vi "校准专用.vi"() -> ()   [LabVIEW 2021]
uses:
  <vilib>/Utility/file.llb/Write Delimited Spreadsheet (DBL).vi
  <vilib>/addons/_NISVFA/_Generation/SoundVib_Generation.lvlib
panel:
  in  "功能选定":u16(ring)=3 items=["保存 10K校准文件", "保存 20K校准文件", "保存 20K无样品文件", "不保存任何文件"]
  out "Time waveform 3":waveform(dbl)(graph)
  out "Time waveform 1":waveform(dbl)(graph)
  out "Time waveform 2":waveform(dbl)(graph)
  out "Time waveform 4":waveform(dbl)(graph)
  in  "开始测量":bool
  in  "停止频率（Hz）":dbl=20000.0 format="%#.2f"
  in  "幅值（V）":dbl=0.1 format="%.3f"
  in  "开始频率（Hz）":dbl=10.0 format="%#.2f"
  # "数据格式：9位小数精度"
  # "注意：\n请确认功能选择正确！\n请把原有文件做好备份再开始测量！新文件会覆盖原有文件。"
  # "扫频激励参数"
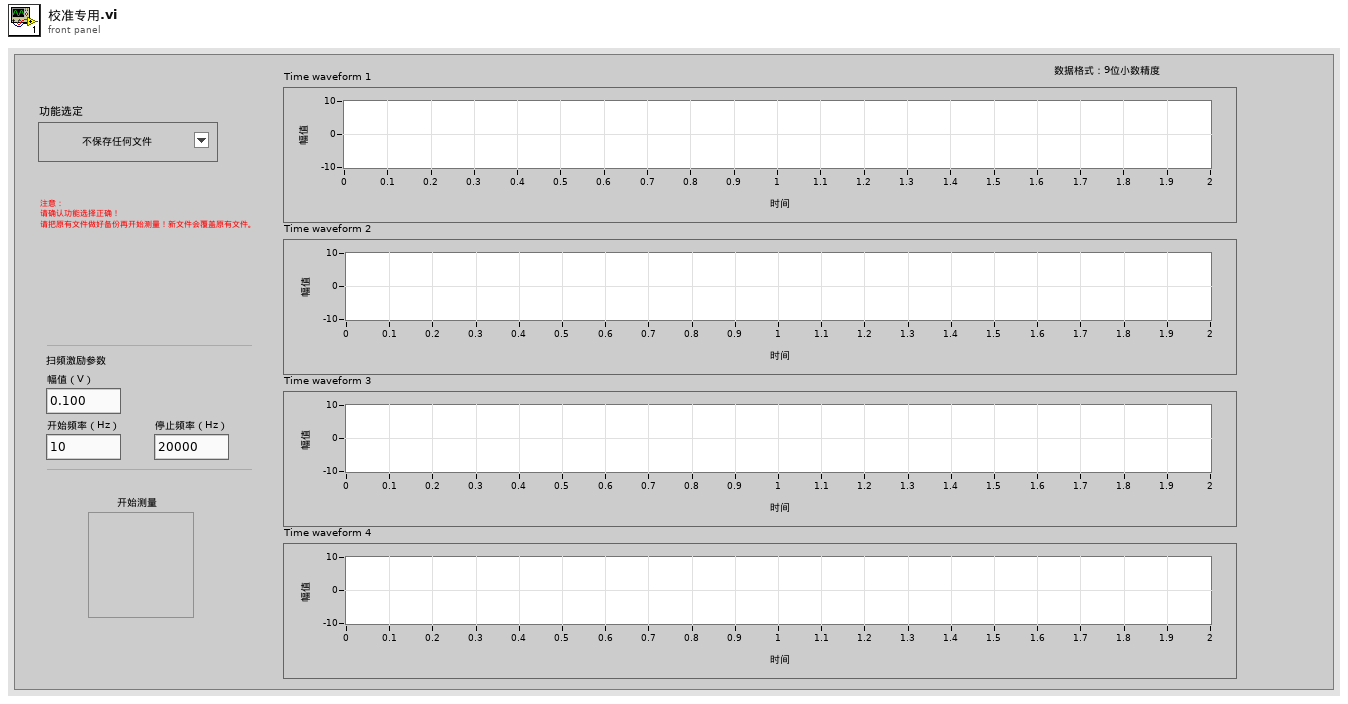
[diagram p1: front panel]
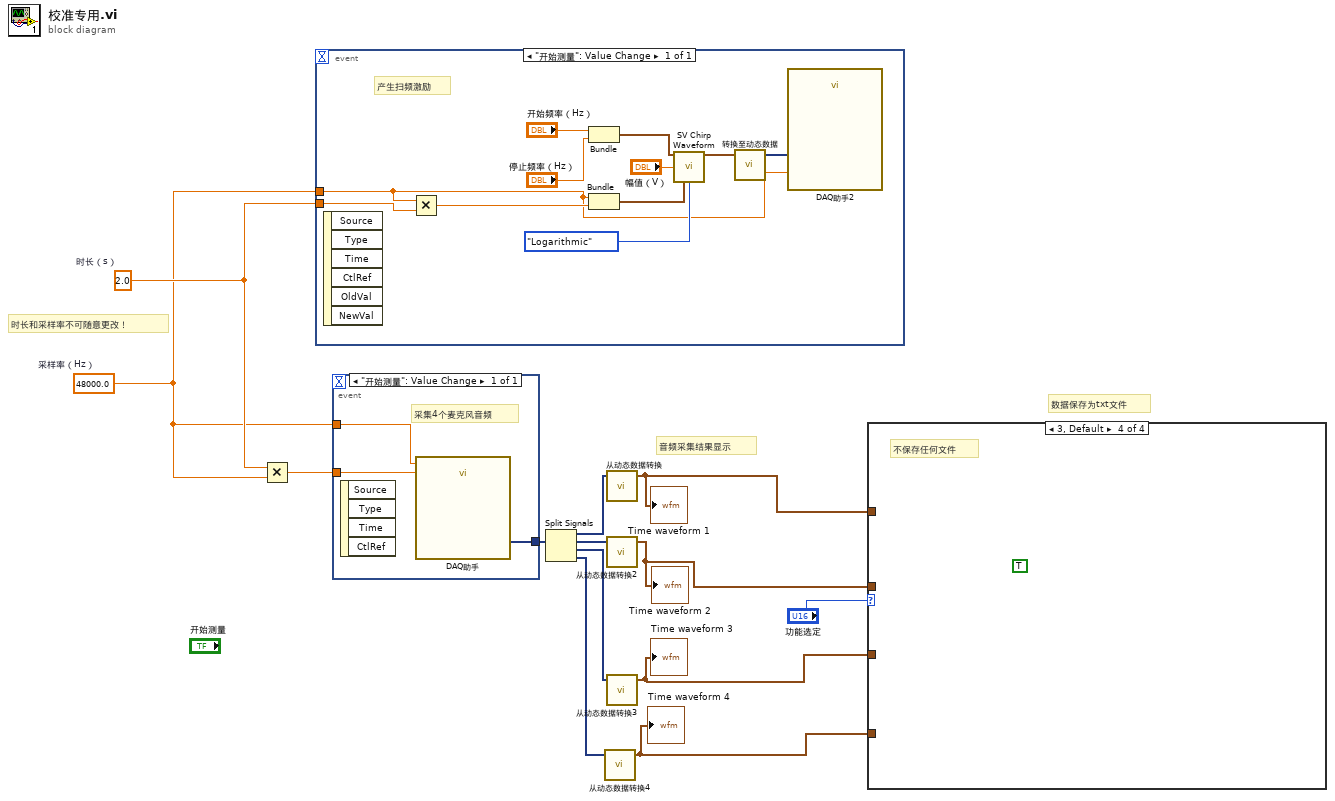
[diagram p0: block diagram]
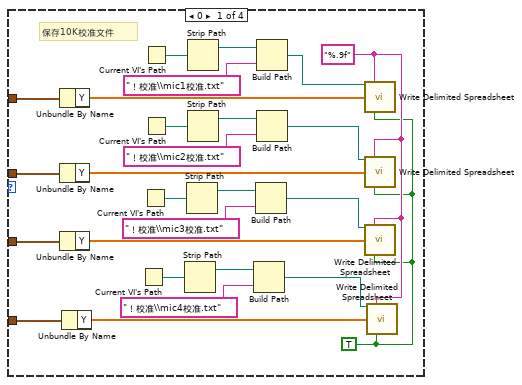
[diagram p2: hidden frame]
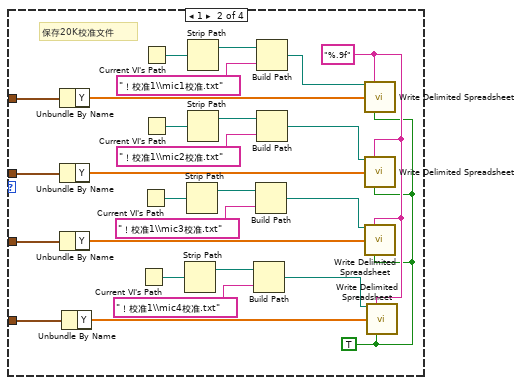
[diagram p3: hidden frame]
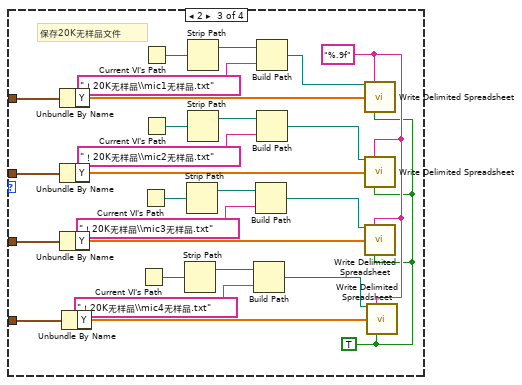
[diagram p4: hidden frame]
diagram:
  w7 = 48000.0  # 采样率（Hz）
  w12 = 2.0  # 时长（s）
  # "数据保存为txt文件"
  # "时长和采样率不可随意更改！"
  # "音频采集结果显示"
  n1 = Multiply(x=w12, y=w7) -> (x*y=w13:dbl)
  n2 = event shown="[0] \"开始测量\": Value Change" {
    selector: _ -> [_]
    dyn-events: _ -> [_]
    timeout: _ -> [_]
    tunnel: w12 -> [w24]
    tunnel: w7 -> [w14]
    event "开始测量": Value Change {
      # "产生扫频激励"
      n3 = event-data() -> ()  [unwired: 1 in, 6 out]
      n4 = Multiply(x=w14, y=w24) -> (x*y=w23:dbl)
      n5 = Bundle("开始频率（Hz）"="开始频率（Hz）", "停止频率（Hz）"="停止频率（Hz）") -> (w16:cluster{"开始频率（Hz）":dbl, "停止频率（Hz）":dbl})  [unwired: 1 in]
      n6 = Bundle("采样率（Hz）"=w14, w23) -> (w21:cluster{"采样率（Hz）":dbl, dbl})  [unwired: 1 in]
      n7 = call <vilib>:"SV Chirp Waveform.vi"("frequency range"=w16, "amplitude"="幅值（V）", "sampling info"=w21, "frequency spacing"=enum16{"Linear", "Logarithmic"}."Logarithmic") -> ("chirp signal"=w22:waveform(dbl))  [unwired: 9 in, 2 out]
      n8 = call "转换至动态数据"("Waveform"=w22) -> ("Dynamic Data Type"=w15:dynamicdata)  [unwired: 3 in]
      n9 = call "DAQ助手2"("data"=w15, "速率"=w14) -> ()  [unwired: 16 in, 2 out]
    }
  }
  n10 = event shown="[0] \"开始测量\": Value Change" {
    selector: _ -> [_]
    dyn-events: _ -> [_]
    timeout: _ -> [_]
    tunnel: [w27] -> w11
    tunnel: w7 -> [w26]
    tunnel: w13 -> [w25]
    event "开始测量": Value Change {
      # "采集4个麦克风音频"
      n11 = event-data() -> ()  [unwired: 1 in, 4 out]
      n12 = call "DAQ助手"("速率"=w26, "采样数"=w25) -> ("data"=w27:dynamicdata)  [unwired: 15 in, 2 out]
    }
  }
  n13 = Split Signals(w11) -> (w8:dynamicdata, w9:dynamicdata, w10:dynamicdata, w6:dynamicdata)  [unwired: 4 in]
  n14 = call "从动态数据转换4"("Dynamic Data Type"=w6) -> ("Waveform"=w2:waveform(dbl))  [unwired: 3 in]
  "Time waveform 4" <- w2
  n15 = call "从动态数据转换"("Dynamic Data Type"=w8) -> ("Waveform"=w5:waveform(dbl))  [unwired: 3 in]
  "Time waveform 1" <- w5
  n16 = call "从动态数据转换2"("Dynamic Data Type"=w9) -> ("Waveform"=w4:waveform(dbl))  [unwired: 3 in]
  "Time waveform 2" <- w4
  n17 = call "从动态数据转换3"("Dynamic Data Type"=w10) -> ("Waveform"=w3:waveform(dbl))  [unwired: 3 in]
  "Time waveform 3" <- w3
  n18 = case shown="3, Default" "功能选定" {
    tunnel: w5 -> [w53 w79 w105 _]
    tunnel: w4 -> [w48 w74 w100 _]
    tunnel: w3 -> [w47 w73 w99 _]
    tunnel: w2 -> [w46 w72 w98 _]
    frame 0 {
      w44 = TRUE ("transpose? (no:F)")
      w45 = "%.9f" ("format (%.3f)")
      # "保存10K校准文件"
      n19 = Unbundle By Name(w53) -> ("Y"=w52:dbl[])
      n20 = Unbundle By Name(w48) -> ("Y"=w51:dbl[])
      n21 = Unbundle By Name(w47) -> ("Y"=w50:dbl[])
      n22 = Unbundle By Name(w46) -> ("Y"=w49:dbl[])
      n23 = Current VI's Path() -> (path=w32:path)
      n24 = Current VI's Path() -> (path=w37:path)
      n25 = Current VI's Path() -> (path=w43:path)
      n26 = Current VI's Path() -> (path=w38:path)
      n27 = Strip Path(path=w32) -> (stripped path=w33:path)  [unwired: 1 out]
      n28 = Strip Path(path=w37) -> (stripped path=w36:path)  [unwired: 1 out]
      n29 = Strip Path(path=w43) -> (stripped path=w42:path)  [unwired: 1 out]
      n30 = Strip Path(path=w38) -> (stripped path=w39:path)  [unwired: 1 out]
      n31 = Build Path(base path=w33, name or relative path="！校准\\mic4校准.txt" ("名称或相对路径")) -> (appended path=w28:path)
      n32 = Build Path(base path=w36, name or relative path="！校准\\mic3校准.txt" ("名称或相对路径")) -> (appended path=w29:path)
      n33 = Build Path(base path=w42, name or relative path="！校准\\mic1校准.txt" ("名称或相对路径")) -> (appended path=w31:path)
      n34 = Build Path(base path=w39, name or relative path="！校准\\mic2校准.txt" ("名称或相对路径")) -> (appended path=w30:path)
      n35 = call-poly <vilib>:"Write Delimited Spreadsheet.vi"("file path (dialog if empty)"=w31, "format (%.3f)"=w45, "1D data"=w52, "transpose? (no:F)"=w44) -> ()  [unwired: 10 in, 2 out]
      n36 = call-poly <vilib>:"Write Delimited Spreadsheet.vi"("file path (dialog if empty)"=w30, "format (%.3f)"=w45, "1D data"=w51, "transpose? (no:F)"=w44) -> ()  [unwired: 10 in, 2 out]
      n37 = call-poly <vilib>:"Write Delimited Spreadsheet.vi"("file path (dialog if empty)"=w29, "format (%.3f)"=w45, "1D data"=w50, "transpose? (no:F)"=w44) -> ()  [unwired: 10 in, 2 out]
      n38 = call-poly <vilib>:"Write Delimited Spreadsheet.vi"("file path (dialog if empty)"=w28, "format (%.3f)"=w45, "1D data"=w49, "transpose? (no:F)"=w44) -> ()  [unwired: 10 in, 2 out]
    }
    frame 1 {
      w70 = TRUE ("transpose? (no:F)")
      w71 = "%.9f" ("format (%.3f)")
      # "保存20K校准文件"
      n39 = Unbundle By Name(w79) -> ("Y"=w78:dbl[])
      n40 = Unbundle By Name(w74) -> ("Y"=w77:dbl[])
      n41 = Unbundle By Name(w73) -> ("Y"=w76:dbl[])
      n42 = Unbundle By Name(w72) -> ("Y"=w75:dbl[])
      n43 = Current VI's Path() -> (path=w58:path)
      n44 = Current VI's Path() -> (path=w63:path)
      n45 = Current VI's Path() -> (path=w69:path)
      n46 = Current VI's Path() -> (path=w64:path)
      n47 = Strip Path(path=w58) -> (stripped path=w59:path)  [unwired: 1 out]
      n48 = Strip Path(path=w63) -> (stripped path=w62:path)  [unwired: 1 out]
      n49 = Strip Path(path=w69) -> (stripped path=w68:path)  [unwired: 1 out]
      n50 = Strip Path(path=w64) -> (stripped path=w65:path)  [unwired: 1 out]
      n51 = Build Path(base path=w59, name or relative path="！校准1\\mic4校准.txt" ("名称或相对路径")) -> (appended path=w54:path)
      n52 = Build Path(base path=w62, name or relative path="！校准1\\mic3校准.txt" ("名称或相对路径")) -> (appended path=w55:path)
      n53 = Build Path(base path=w68, name or relative path="！校准1\\mic1校准.txt" ("名称或相对路径")) -> (appended path=w57:path)
      n54 = Build Path(base path=w65, name or relative path="！校准1\\mic2校准.txt" ("名称或相对路径")) -> (appended path=w56:path)
      n55 = call-poly <vilib>:"Write Delimited Spreadsheet.vi"("file path (dialog if empty)"=w57, "format (%.3f)"=w71, "1D data"=w78, "transpose? (no:F)"=w70) -> ()  [unwired: 10 in, 2 out]
      n56 = call-poly <vilib>:"Write Delimited Spreadsheet.vi"("file path (dialog if empty)"=w56, "format (%.3f)"=w71, "1D data"=w77, "transpose? (no:F)"=w70) -> ()  [unwired: 10 in, 2 out]
      n57 = call-poly <vilib>:"Write Delimited Spreadsheet.vi"("file path (dialog if empty)"=w55, "format (%.3f)"=w71, "1D data"=w76, "transpose? (no:F)"=w70) -> ()  [unwired: 10 in, 2 out]
      n58 = call-poly <vilib>:"Write Delimited Spreadsheet.vi"("file path (dialog if empty)"=w54, "format (%.3f)"=w71, "1D data"=w75, "transpose? (no:F)"=w70) -> ()  [unwired: 10 in, 2 out]
    }
    frame 2 {
      w96 = TRUE ("transpose? (no:F)")
      w97 = "%.9f" ("format (%.3f)")
      # "保存20K无样品文件"
      n59 = Unbundle By Name(w105) -> ("Y"=w104:dbl[])
      n60 = Unbundle By Name(w100) -> ("Y"=w103:dbl[])
      n61 = Unbundle By Name(w99) -> ("Y"=w102:dbl[])
      n62 = Unbundle By Name(w98) -> ("Y"=w101:dbl[])
      n63 = Current VI's Path() -> (path=w84:path)
      n64 = Current VI's Path() -> (path=w89:path)
      n65 = Current VI's Path() -> (path=w95:path)
      n66 = Current VI's Path() -> (path=w90:path)
      n67 = Strip Path(path=w84) -> (stripped path=w85:path)  [unwired: 1 out]
      n68 = Strip Path(path=w89) -> (stripped path=w88:path)  [unwired: 1 out]
      n69 = Strip Path(path=w95) -> (stripped path=w94:path)  [unwired: 1 out]
      n70 = Strip Path(path=w90) -> (stripped path=w91:path)  [unwired: 1 out]
      n71 = Build Path(base path=w85, name or relative path="！20K无样品\\mic4无样品.txt" ("名称或相对路径")) -> (appended path=w80:path)
      n72 = Build Path(base path=w88, name or relative path="！20K无样品\\mic3无样品.txt" ("名称或相对路径")) -> (appended path=w81:path)
      n73 = Build Path(base path=w94, name or relative path="！20K无样品\\mic1无样品.txt" ("名称或相对路径")) -> (appended path=w83:path)
      n74 = Build Path(base path=w91, name or relative path="！20K无样品\\mic2无样品.txt" ("名称或相对路径")) -> (appended path=w82:path)
      n75 = call-poly <vilib>:"Write Delimited Spreadsheet.vi"("file path (dialog if empty)"=w83, "format (%.3f)"=w97, "1D data"=w104, "transpose? (no:F)"=w96) -> ()  [unwired: 10 in, 2 out]
      n76 = call-poly <vilib>:"Write Delimited Spreadsheet.vi"("file path (dialog if empty)"=w82, "format (%.3f)"=w97, "1D data"=w103, "transpose? (no:F)"=w96) -> ()  [unwired: 10 in, 2 out]
      n77 = call-poly <vilib>:"Write Delimited Spreadsheet.vi"("file path (dialog if empty)"=w81, "format (%.3f)"=w97, "1D data"=w102, "transpose? (no:F)"=w96) -> ()  [unwired: 10 in, 2 out]
      n78 = call-poly <vilib>:"Write Delimited Spreadsheet.vi"("file path (dialog if empty)"=w80, "format (%.3f)"=w97, "1D data"=w101, "transpose? (no:F)"=w96) -> ()  [unwired: 10 in, 2 out]
    }
    frame 3, Default {
      (unwired) TRUE
      # "不保存任何文件"
    }
  }
